vi "GetCals.vi"   [LabVIEW 2019]
uses:
  <vilib>/Utility/file.llb/Read Delimited Spreadsheet (string).vi
  <vilib>/Rock Robotics/Network Tables/NT Write String Array.vi
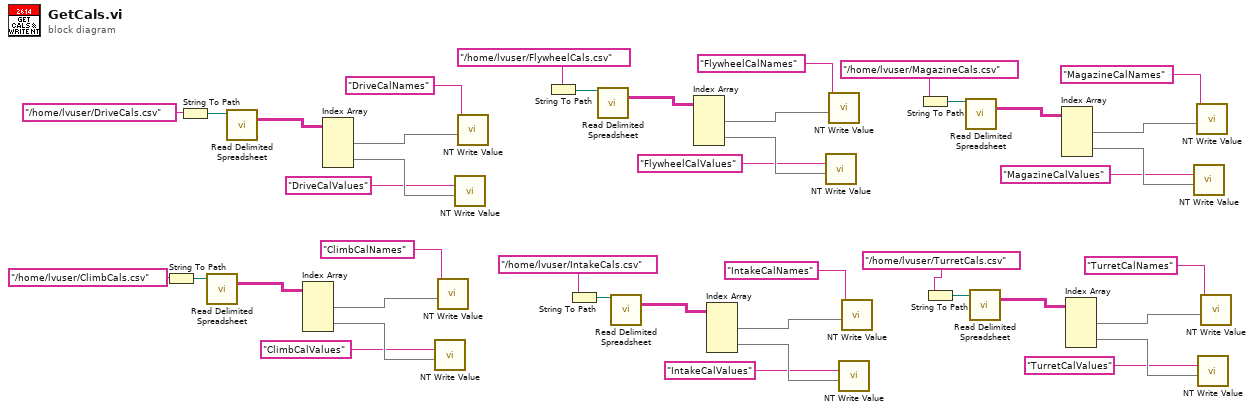
[diagram p0: block diagram]
diagram:
  n1 = String To Path(string="/home/lvuser/ClimbCals.csv") -> (path=w9:path)
  n2 = String To Path(string="/home/lvuser/DriveCals.csv") -> (path=w11:path)
  n3 = call-poly <vilib>:"Read Delimited Spreadsheet.vi"("file path (dialog if empty)"=w9) -> ("all rows"=w37:string[][])  [unwired: 9 in, 5 out]
  n4 = call-poly <vilib>:"Read Delimited Spreadsheet.vi"("file path (dialog if empty)"=w11) -> ("all rows"=w42:string[][])  [unwired: 9 in, 5 out]
  n5 = Index Array(array=w37) -> (element #1=w35:string[], element #2=w36:string[])  [unwired: 4 in]
  n6 = Index Array(array=w42) -> (element #1=w40:string[], element #2=w41:string[])  [unwired: 4 in]
  n7 = call-poly <vilib>:"NT Write Value.vi"("String Array"=w36, "Name"="ClimbCalValues") -> ()  [unwired: 9 in, 1 out]
  n8 = call-poly <vilib>:"NT Write Value.vi"("String Array"=w35, "Name"="ClimbCalNames") -> ()  [unwired: 9 in, 1 out]
  n9 = call-poly <vilib>:"NT Write Value.vi"("String Array"=w41, "Name"="DriveCalValues") -> ()  [unwired: 9 in, 1 out]
  n10 = call-poly <vilib>:"NT Write Value.vi"("String Array"=w40, "Name"="DriveCalNames") -> ()  [unwired: 9 in, 1 out]
  n11 = String To Path(string="/home/lvuser/FlywheelCals.csv") -> (path=w7:path)
  n12 = String To Path(string="/home/lvuser/IntakeCals.csv") -> (path=w5:path)
  n13 = call-poly <vilib>:"Read Delimited Spreadsheet.vi"("file path (dialog if empty)"=w7) -> ("all rows"=w32:string[][])  [unwired: 9 in, 5 out]
  n14 = call-poly <vilib>:"Read Delimited Spreadsheet.vi"("file path (dialog if empty)"=w5) -> ("all rows"=w27:string[][])  [unwired: 9 in, 5 out]
  n15 = Index Array(array=w32) -> (element #1=w30:string[], element #2=w31:string[])  [unwired: 4 in]
  n16 = Index Array(array=w27) -> (element #1=w25:string[], element #2=w26:string[])  [unwired: 4 in]
  n17 = call-poly <vilib>:"NT Write Value.vi"("String Array"=w31, "Name"="FlywheelCalValues") -> ()  [unwired: 9 in, 1 out]
  n18 = call-poly <vilib>:"NT Write Value.vi"("String Array"=w30, "Name"="FlywheelCalNames") -> ()  [unwired: 9 in, 1 out]
  n19 = call-poly <vilib>:"NT Write Value.vi"("String Array"=w26, "Name"="IntakeCalValues") -> ()  [unwired: 9 in, 1 out]
  n20 = call-poly <vilib>:"NT Write Value.vi"("String Array"=w25, "Name"="IntakeCalNames") -> ()  [unwired: 9 in, 1 out]
  n21 = String To Path(string="/home/lvuser/MagazineCals.csv") -> (path=w3:path)
  n22 = String To Path(string="/home/lvuser/TurretCals.csv") -> (path=w1:path)
  n23 = call-poly <vilib>:"Read Delimited Spreadsheet.vi"("file path (dialog if empty)"=w3) -> ("all rows"=w22:string[][])  [unwired: 9 in, 5 out]
  n24 = call-poly <vilib>:"Read Delimited Spreadsheet.vi"("file path (dialog if empty)"=w1) -> ("all rows"=w17:string[][])  [unwired: 9 in, 5 out]
  n25 = Index Array(array=w22) -> (element #1=w20:string[], element #2=w21:string[])  [unwired: 4 in]
  n26 = Index Array(array=w17) -> (element #1=w15:string[], element #2=w16:string[])  [unwired: 4 in]
  n27 = call-poly <vilib>:"NT Write Value.vi"("String Array"=w21, "Name"="MagazineCalValues") -> ()  [unwired: 9 in, 1 out]
  n28 = call-poly <vilib>:"NT Write Value.vi"("String Array"=w20, "Name"="MagazineCalNames") -> ()  [unwired: 9 in, 1 out]
  n29 = call-poly <vilib>:"NT Write Value.vi"("String Array"=w16, "Name"="TurretCalValues") -> ()  [unwired: 9 in, 1 out]
  n30 = call-poly <vilib>:"NT Write Value.vi"("String Array"=w15, "Name"="TurretCalNames") -> ()  [unwired: 9 in, 1 out]
